vi "DownloadFile.vi"(5 "Latest runtime":T1, 6 "error in":errorcluster, 9 "Download Folder":path) -> (0 "error out":errorcluster, 3 "file":path)   [LabVIEW 2014, in "GitHub API.lvlib"]
uses:
  GitHub API.lvlib
  TypeDefs/GitHubContents_TD.ctl
  <vilib>/httpClient/LabVIEWHTTPClient.lvlib
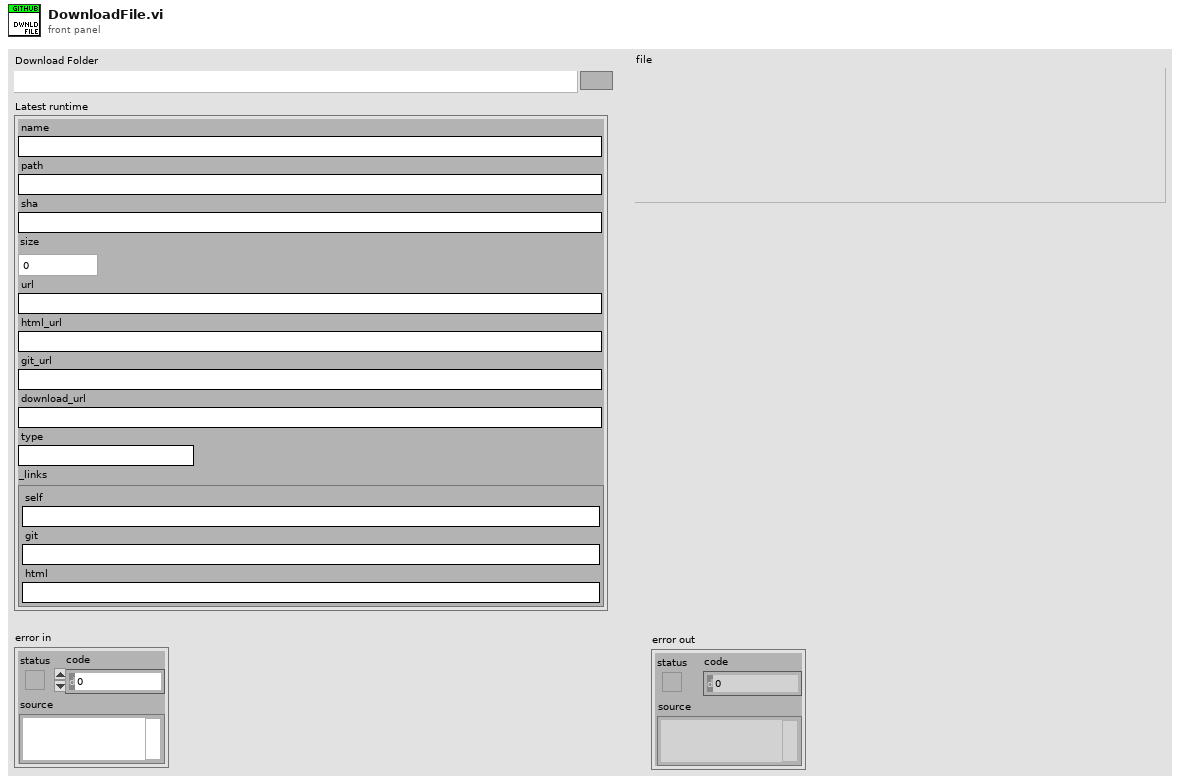
[diagram p1: front panel]
types:
  T1 = typedef "GitHub API.lvlib/GitHubContents_TD.ctl" = cluster{"name":string, "path":string, "sha":string, "size":dbl, "url":string, "html_url":string, "git_url":string, "download_url":string, "type":string, "_links":cluster{"self":string, "git":string, "html":string}}
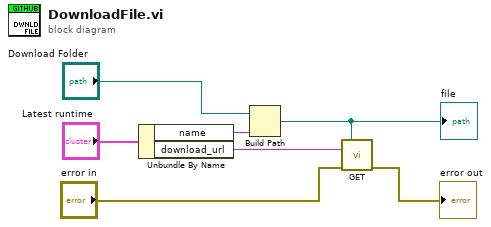
[diagram p0: block diagram]
diagram:
  n1 = Unbundle By Name("Latest runtime") -> ("name"=w5:string, "download_url"=w6:string)
  n2 = Build Path(base path="Download Folder", name or relative path=w5) -> (appended path=w2:path)
  "file" <- w2
  n3 = call <vilib>:"GET.vi"("output file"=w2, "url"=w6, "error in (no error)"="error in") -> ("error out"=→"error out":errorcluster)  [unwired: 9 in, 3 out]
